vi "runtime io test.vi"() -> ()   [LabVIEW 2014, in "Simple Sequencer TBM tests.lvlib"]
uses:
  <vilib>/NI/TBM Modules/Sequencer/testing/Simple Sequencer TBM tests.lvlib
  <vilib>/NI/TBM Modules/Sequencer/module/execution/Simple Sequencer TBM runtime.lvclass
  <vilib>/NI/TBM Modules/Sequencer/module/configuration/Simple Sequencer TBM configuration.lvclass
  <vilib>/NI/Tag Bus/dictionary/data dictionary.lvclass
  <vilib>/NI/Tag Bus/dictionary/lookup polymorphs/locate double.vi
  <vilib>/NI/Tag Bus Module Framework/channel/TBM channel.lvclass
  <vilib>/NI/Tag Bus/table/data table.lvlib
  <vilib>/NI/Tag Bus/table/data polymorphs/write one/write Double.vi
panel:
  out "results set":bool
  out "no error":errorcluster
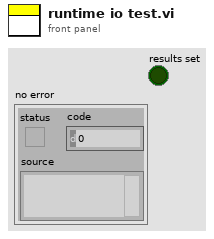
[diagram p1: front panel]
types:
  T1 = typedef "TBM channel.lvclass/data tables.ctl" = cluster{"input data":T2, "processing parameter":T2, "processing result":T2, "output data":T2}
  T2 = typedef "tag bus.lvlib/dictionary table pair.ctl" = cluster{"data dictionary":refnum<class "data dictionary.lvclass">, "data table":T3}
  T3 = typedef "tag bus.lvlib/data table.lvlib/data table.ctl" = cluster{"Double":dbl[], "Single":sgl[], "I64":i64[], "I32":i32[], "I16":i16[], "I8":i8[], "U64":u64[], "U32":u32[], "U16":u16[], "U8":u8[], "Boolean":bool[], "String":string[], "Array of Double":cluster{"DBL Array":dbl[]}[], "Array of Single":cluster{"SGL Array":sgl[]}[], "Array of I64":cluster{"I64 Array":i64[]}[], "Array of I32":cluster{"I32 Array":i32[]}[], "Array of I16":cluster{"I16 Array":i16[]}[], "Array of I8":cluster{"I8 Array":i8[]}[], "Array of U64":cluster{"U64 Array":u64[]}[], "Array of U32":cluster{"U32 Array":u32[]}[], "Array of U16":cluster{"U16 Array":u16[]}[], "Array of U8":cluster{"U8 Array":u8[]}[], "Array of Boolean":cluster{"Boolean Array":bool[]}[], "Array of String":cluster{"String Array":string[]}[]}
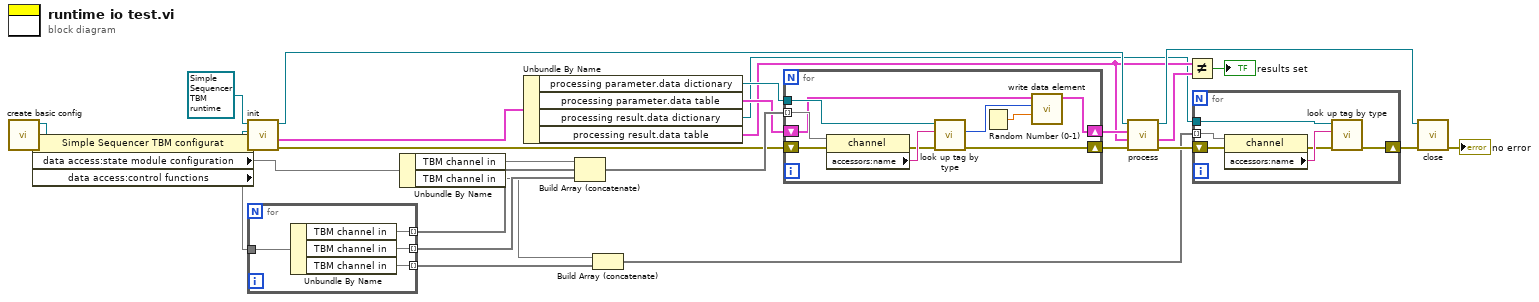
[diagram p0: block diagram]
diagram:
  n1 = call <vilib>:"create basic config.vi"() -> ("error out"=w26:errorcluster, "user tag bus module configuration out"=w24:refnum<class "Simple Sequencer TBM configuration.lvclass">)  [unwired: 8 in, 2 out]
  n2 = property class="Simple Sequencer TBM configurat"(reference=w24, error in=w26) -> (reference out=w23:refnum<class "Simple Sequencer TBM configuration.lvclass">, error out=w25:errorcluster, "data access:state module configuration"=w22, "data access:control functions"=w20)
  n3 = call-dynamic "init.vi"("error in"=w25, "module configuration"=w23, "Simple Sequencer TBM runtime in"=refnum<class "Simple Sequencer TBM runtime.lvclass"> refnum ("tag bus configurable plugin module")) -> ("error out"=w11:errorcluster, "data allocations"=w28:T1, "Simple Sequencer TBM runtime out"=w21:refnum<class "Simple Sequencer TBM runtime.lvclass">)  [unwired: 5 in, 1 out]
  n4 = for {
    tunnel: w20 -> [w33]
    tunnel: [w32] -> w18 mode=indexing
    tunnel: [w31] -> w17 mode=indexing
    tunnel: [w30] -> w16 mode=indexing
    n5 = Unbundle By Name(w33) -> ("TBM channel in"=w32, "TBM channel in"=w31, "TBM channel in"=w30)
  }
  n6 = Unbundle By Name(w22) -> ("TBM channel in"=w19, "TBM channel in"=w15)
  n7 = Unbundle By Name(w28) -> ("processing parameter.data dictionary"=w14:refnum<class "data dictionary.lvclass">, "processing parameter.data table"=w10:T3, "processing result.data dictionary"=w1:refnum<class "data dictionary.lvclass">, "processing result.data table"=w4:T3)
  n8 = Build Array (concatenate)(w19, w18, w17) -> (w13:void[])
  n9 = Build Array (concatenate)(w15, w16) -> (w2:void[])
  n10 = for {
    tunnel: w14 -> [w43]
    tunnel: w13 -> [w42] mode=indexing
    shift-right: [w39] -> w12
    shift-left: w11 -> [w38]
    shift-right: [w36] -> w9
    shift-left: w10 -> [w37]
    n11 = property class="channel"(reference=w42, error in=w38) -> (error out=w40:errorcluster, "accessors:name"=w41:string)  [unwired: 1 out]
    n12 = call-poly <vilib>:"look up tag by type.vi"("error in"=w40, "name"=w41, "data dictionary in"=w43) -> ("error out"=w39:errorcluster, "index"=w35:i32)  [unwired: 6 in, 1 out]
    n13 = Random Number (0-1)() -> (number: 0 to 1=w34:dbl)
    n14 = call-poly <vilib>:"write data element.vi"("value"=w34, "index"=w35, "data table in"=w37) -> ("data table out"=w36:T3)  [unwired: 8 in]
  }
  n15 = call-dynamic "process.vi"("error in"=w12, "result allocation"=w4, "parameters"=w9, "Simple Sequencer TBM runtime in"=w21) -> ("error out"=w7:errorcluster, "results"=w5:T3, "Simple Sequencer TBM runtime out"=w8:refnum<class "Simple Sequencer TBM runtime.lvclass">)  [unwired: 4 in, 1 out]
  n16 = Not Equal?(x=w4, y=w5) -> (x != y?=→"results set":bool)
  n17 = for {
    tunnel: w2 -> [w49] mode=indexing
    shift-right: [w46] -> w6
    shift-left: w7 -> [w45]
    tunnel: w1 -> [w44]
    n18 = property class="channel"(reference=w49, error in=w45) -> (error out=w47:errorcluster, "accessors:name"=w48:string)  [unwired: 1 out]
    n19 = call-poly <vilib>:"look up tag by type.vi"("error in"=w47, "name"=w48, "data dictionary in"=w44) -> ("error out"=w46:errorcluster)  [unwired: 6 in, 2 out]
  }
  n20 = call-dynamic "close.vi"("error in"=w6, "Simple Sequencer TBM runtime in"=w8) -> ("error out"=→"no error":errorcluster)  [unwired: 9 in]
